vi "Check 24 Hrs Passed.vi"(9 "Time String":string, 11 "Date String":string) -> (3 "24 Hrs Passed?":bool)   [LabVIEW 2018]
uses:
  <vilib>/Utility/miscctls.llb/LVDateTimeRec.ctl
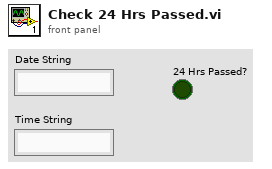
[diagram p1: front panel]
types:
  T1 = typedef "LVDateTimeRec.ctl" = cluster{"fractional second":dbl, "second":i32, "minute":i32, "hour":i32, "day of month":i32, "month":i32, "year":i32, "day of week":i32, "day of year":i32, "DST":i32}
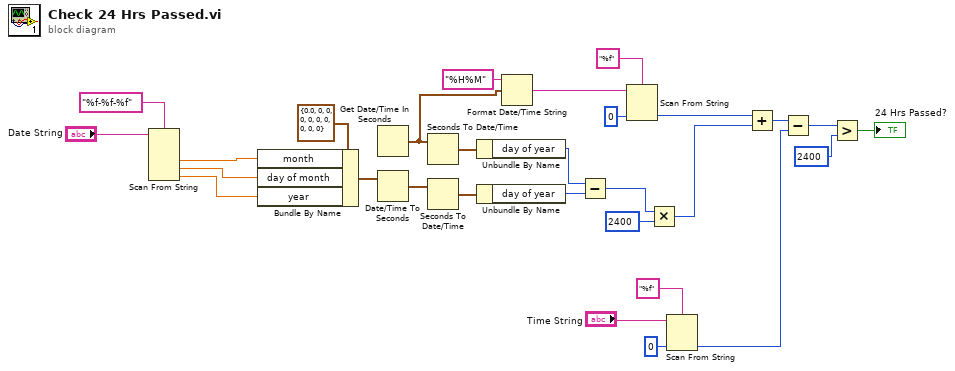
[diagram p0: block diagram]
diagram:
  n1 = Scan From String(format string="%f-%f-%f", input string="Date String") -> (output 1=w27:dbl, output 2=w23:dbl, output 3=w26:dbl)  [unwired: 5 in, 3 out]
  n2 = Bundle By Name(cluster=T1 {"fractional second"=0.0, "second"=0, "minute"=0, "hour"=0, "day of month"=0, "month"=0, "year"=0, "day of week"=0, "day of year"=0, "DST"=0} ("date time rec"), "month"=w27, "day of month"=w23, "year"=w26) -> (w24:T1)
  n3 = Get Date/Time In Seconds() -> (seconds since 1Jan1904=w11:timestamp)
  n4 = Date/Time To Seconds(2:w24) -> (0:w21:timestamp)  [unwired: 1 in]
  n5 = Seconds To Date/Time(time stamp (now)=w11) -> (date time rec=w22:T1)  [unwired: 1 in]
  n6 = Seconds To Date/Time(time stamp (now)=w21) -> (date time rec=w20:T1)  [unwired: 1 in]
  n7 = Unbundle By Name(w22) -> ("day of year"=w18:i32)
  n8 = Unbundle By Name(w20) -> ("day of year"=w19:i32)
  n9 = Format Date/Time String(time format string (%c)="%H%M", seconds (now)=w11) -> (date/time string=w8:string)  [unwired: 1 in]
  n10 = Subtract(x=w18, y=w19) -> (x-y=w17:i32)
  n11 = Scan From String(format string="%f", input string=w8, default 1=0 ("default value 1")) -> (output 1=w7:i32)  [unwired: 2 in, 3 out]
  n12 = Multiply(x=w17, y=2400) -> (x*y=w6:i32)
  n13 = Scan From String(format string="%f", input string="Time String", default 1=0 ("default value 1")) -> (output 1=w5:i32)  [unwired: 2 in, 3 out]
  n14 = Add(x=w7, y=w6) -> (x+y=w4:i32)
  n15 = Subtract(x=w4, y=w5) -> (x-y=w3:i32)
  n16 = Greater?(x=w3, y=2400) -> (0:→"24 Hrs Passed?":bool)
